vi "Dichtheitstest speichern.vi"   [LabVIEW 2020, in "Erweiterte Konfig.lvlib"]
uses:
  Erweiterte Konfig.lvlib
  Funktionstasten/Funktionstasten-Aktion.ctl
  Funktionstasten/Zustaende.ctl
  Sprachverwaltung/FGV Aktion Tabelle zerlegen.ctl
  Allgemein/allgemeine Sub-VIs.lvlib
  Sprachverwaltung/Sprachverwaltung.lvlib
  Linearisierung V2/Protokoll/Protokoll.lvlib
  Funktionstasten/Funktionstasten.lvlib
types:
  T1 = typedef "Funktionstasten.lvlib/Zustaende.ctl" = enum16{"Standby", "Pause", "Eco", "Messen", "Kalibrieren", "Spülen Filter", "Spülen Leitung", "Umgebungsluft", "0-Gas", "Cal-Gas", "CG zu PNS", "-------------", "Init 1", "Init 2", "Init 3", "Init 4", "Messen vorbereiten", "Messen durchführen", "Exit"}
  T2 = typedef "Funktionstasten.lvlib/Funktionstasten-Aktion.ctl" = enum16{"Initialisieren", "Zustand setzen", "Taste gedrückt", "Fehler speichern", "Lesen", "Manuell", "Remote", "Bitparallel", "Samplepoint", "Zeit Prüfen", "reset Umschalten"}
  T3 = typedef "Sprachverwaltung.lvlib/FGV Aktion Tabelle zerlegen.ctl" = enum16{"laden", "vereinzeln", "speichern"}
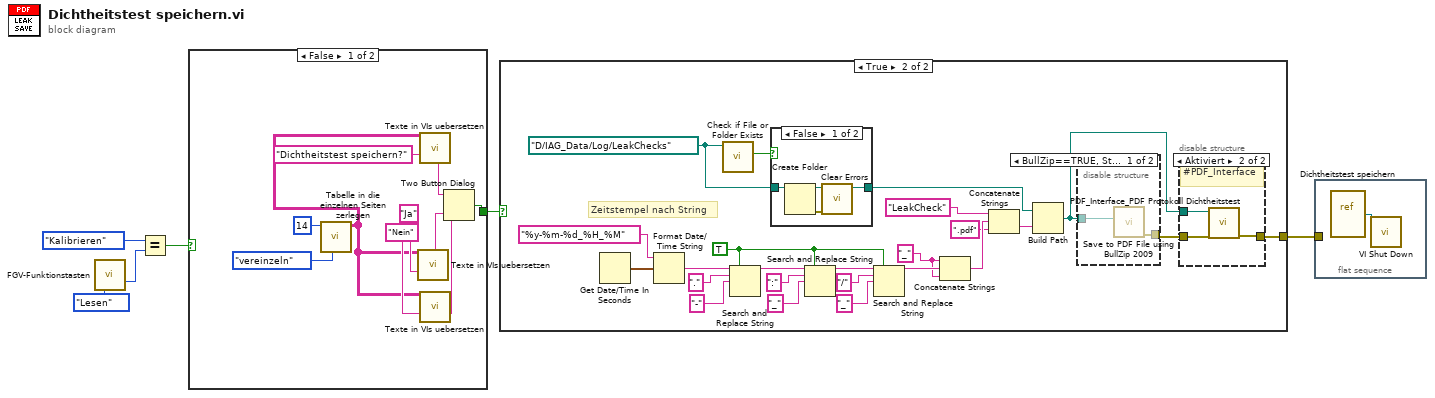
[diagram p0: block diagram]
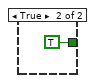
[diagram p2: hidden frame]
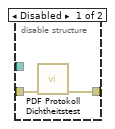
[diagram p4: hidden frame]
diagram:
  n1 = call "FGV-Funktionstasten.vi"("Aktion"=Funktionstasten-Aktion."Lesen") -> ("ausgewählte Funktion"=w3:T1)  [unwired: 7 in, 7 out]
  n2 = Equal?(x=Zustaende."Kalibrieren", y=w3) -> (x = y?=w1:bool)
  n3 = case shown="False" w1 {
    tunnel: [w7 TRUE ("T button?")] -> w5
    frame False {
      n4 = call "Tabelle in die einzelnen Seiten zerlegen.vi"("Aktion"=FGV_Aktion_Tabelle_zerlegen."vereinzeln", "Index (Seite)"=14) -> ("Sprachliste"=w8:string[][])  [unwired: 7 in, 2 out]
      n5 = call "Texte in VIs uebersetzen.vi"("Sprachliste"=w8, "String zum Übersetzen"="Ja" ("Text für T-Schaltfläche (\"OK\")")) -> ("String zum Übersetzen"=w11:string)  [unwired: 9 in, 4 out]
      n6 = call "Texte in VIs uebersetzen.vi"("Sprachliste"=w8, "String zum Übersetzen"="Dichtheitstest speichern?" ("Nachricht")) -> ("String zum Übersetzen"=w13:string)  [unwired: 9 in, 4 out]
      n7 = call "Texte in VIs uebersetzen.vi"("Sprachliste"=w8, "String zum Übersetzen"="Nein" ("Text für F-Schaltfläche (\"Abbrechen\")")) -> ("String zum Übersetzen"=w9:string)  [unwired: 9 in, 4 out]
      n8 = Two Button Dialog(message=w13, 1:w9, 2:w11) -> (T button?=w7:bool)
    }
    frame True {
    }
  }
  n9 = case shown="True" w5 {
    tunnel: [_ w41] -> w6
    frame False {
    }
    frame True {
      w19 = "_"
      w31 = TRUE ("Alle ersetzen? (F)")
      w23 = path "D:/IAG_Data/Log/LeakChecks" ("Grundpfad")
      # "Zeitstempel nach String"
      n10 = Get Date/Time In Seconds() -> (seconds since 1Jan1904=w35:timestamp)
      n11 = Format Date/Time String(time format string (%c)="%y-%m-%d_%H_%M" ("Zeitformatierungs-String (%c)"), seconds (now)=w35) -> (date/time string=w36:string)  [unwired: 1 in]
      n12 = call <vilib>:"Check if File or Folder Exists.vi"("path"=w23) -> ("file or folder exists?"=w33:bool)  [unwired: 8 in, 2 out]
      n13 = Search and Replace String(replace all?=w31, input string=w36, search string="." ("Such-String"), replace string="-" ("String ersetzen(\"\")")) -> (result string=w37:string)  [unwired: 4 in, 3 out]
      n14 = case shown="False" w33 {
        tunnel: w23 -> [w51 w52]
        tunnel: [w49 w52] -> w34
        frame False {
          n15 = Create Folder(path (use dialog)=w51) -> (created path=w49:path, error out=w50:errorcluster)  [unwired: 2 in, 1 out]
          n16 = call <vilib>:"Clear Errors.vi"("error in (no error)"=w50) -> ()  [unwired: 5 in, 2 out]
        }
        frame True {
        }
      }
      n17 = Search and Replace String(replace all?=w31, input string=w37, search string=":" ("Such-String"), replace string="_" ("String ersetzen(\"\")")) -> (result string=w38:string)  [unwired: 4 in, 3 out]
      n18 = Search and Replace String(replace all?=w31, input string=w38, search string="/" ("Such-String"), replace string="_" ("String ersetzen(\"\")")) -> (result string=w39:string)  [unwired: 4 in, 3 out]
      n19 = Concatenate Strings(w19, w39, w19) -> (w40:string)
      n20 = Concatenate Strings("LeakCheck" ("String"), w40, ".pdf") -> (w32:string)
      n21 = Build Path(base path=w34, name or relative path=w32) -> (appended path=w18:path)
      n22 = disable-structure shown="BullZip==TRUE, Standard" {
        disable-tunnel: w18 -> [w48 _]
        disable-tunnel: [w47 _] -> w20
        frame condition #0 {
          n23 = call "Save to PDF File using BullZip 2009.vi"("Save PDF File Path"=w48) -> ("error out"=w47:errorcluster)  [unwired: 10 in]
        }
        frame condition #1 (active) {
        }
      }
      n24 = disable-structure shown="Aktiviert" {
        disable-tunnel: [w43 w45] -> w41
        disable-tunnel: w20 -> [w42 w46]
        disable-tunnel: w18 -> [_ w44]
        frame Disabled {
          n25 = call "PDF Protokoll Dichtheitstest.vi"("error in (no error)"=w42) -> ("error out"=w43:errorcluster)  [unwired: 10 in]
        }
        frame Enabled {
          # "#PDF_Interface"
          n26 = call "PDF_Interface_PDF Protokoll Dichtheitstest.vi"("error in (no error)"=w46, "Save PDF File Path"=w44) -> ("error out"=w45:errorcluster)  [unwired: 9 in]
        }
      }
    }
  }
  n27 = flat-sequence {
    tunnel: w6 -> [_]
    frame #0 {
      n28 = vi-ref "Dichtheitstest speichern.vi"() -> (w53:refnum<vi>)
      n29 = call "VI Shut Down.vi"("VI Referenz"=w53) -> ()  [unwired: 11 in]
    }
  }
